vi "poly_eval.vi"(2 "P(x)":dbl[](array[numeric]) min=0.0 max=127.0 format="%#.2f", 3 "A":dbl) -> (1 "P(A)":dbl)   [LabVIEW 2020]
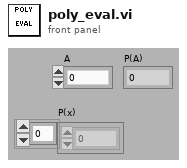
[diagram p1: front panel]
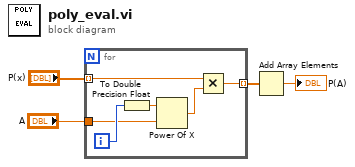
[diagram p0: block diagram]
diagram:
  n1 = for {
    tunnel: "P(x)" -> [w7] mode=indexing
    tunnel: [w8] -> w1 mode=indexing
    tunnel: "A" -> [w5]
    i -> [w10]
    n2 = To Double Precision Float(number=w10) -> (double precision float=w6:dbl)
    n3 = Power Of X(1:w5, 2:w6) -> (0:w9:dbl)
    n4 = Multiply(x=w7, y=w9) -> (x*y=w8:dbl)
  }
  n5 = Add Array Elements(numeric array=w1) -> (sum=→"P(A)":dbl)
